vi "GUI.vi"() -> ()   [LabVIEW 2023]
uses:
  <vilib>/Platform/TimedLoop/XDataNode/timing_clust.ctl
  <vilib>/Platform/TimedLoop/XDataNode/nitl_modes.ctl
  <vilib>/Platform/TimedLoop/XDataNode/wakeup.ctl
  <vilib>/Instr/_visa.llb/VISA Configure Serial Port (Instr).vi
  <vilib>/Platform/TimedLoop/XDataNode/XDataNode.xnode
  <vilib>/Platform/TimedLoop/XDataNode/XDNodeRunTimeDep.lvlib
panel:
  out "read buffer":string
  out "Duty":sgl format="%#.4f"
  in  "?":bool
  in  "KD":sgl=0.001 format="%#.4f"
  in  "KI":sgl=0.1 format="%#.4f"
  in  "KP":sgl=1.0 format="%#.4f"
  out "Actual speed":sgl format="%#.1g"
  out "Actual speed":sgl(slide) scale=0.0..3000.0
  out "REV":bool
  out "FWD":bool
  in  "?":bool
  in  "Controller port":refnum<visa-resource-name>
  out "Actual set speed":sgl format="%#.1g"
  out "Throttle set speed":sgl format="%#.0f"
  out "?":T1(graph)
  out "Actual set speed":sgl(slide) scale=0.0..3000.0
  out "Throttle set speed":sgl(slide) scale=0.0..3000.0
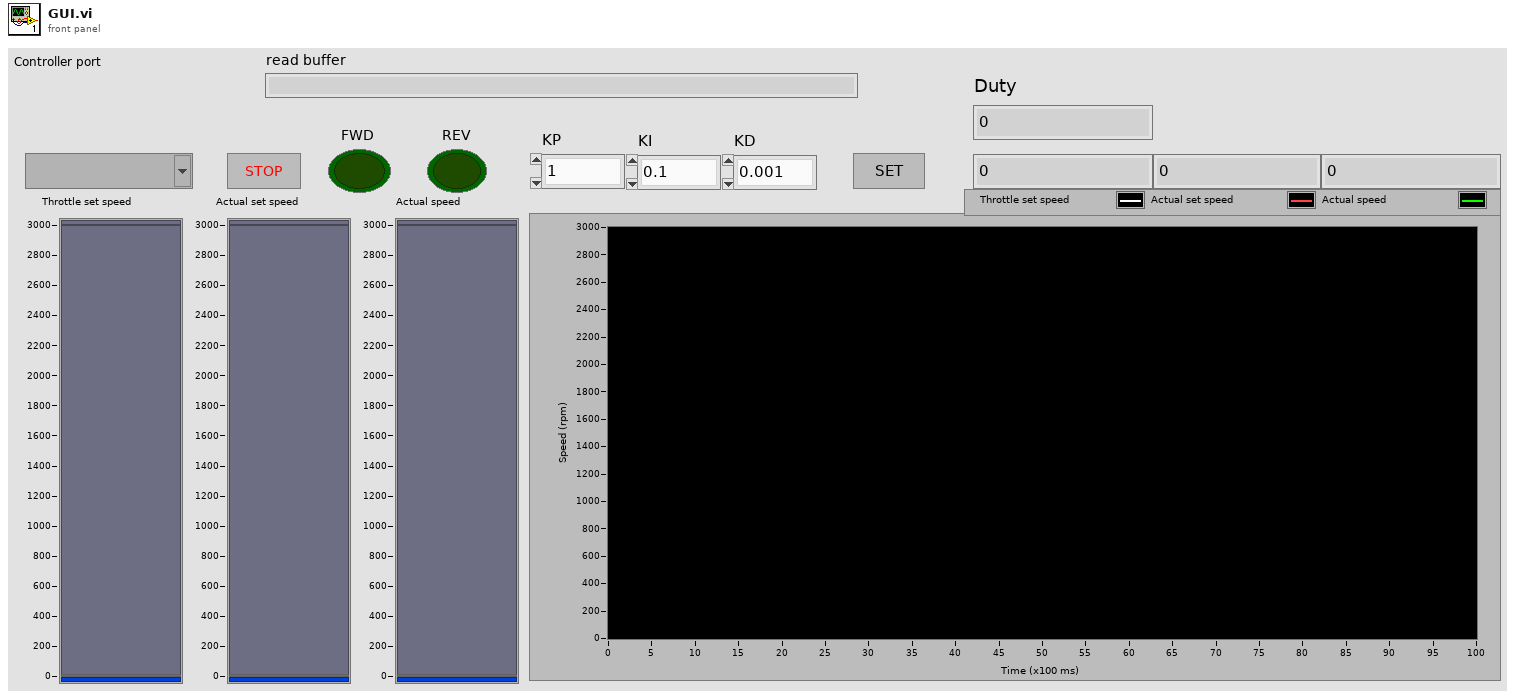
[diagram p1: front panel]
types:
  T1 = cluster{"num_float":sgl, "num_float":sgl, "num_float":sgl}
  T2 = typedef "XDNodeRunTimeDep.lvlib/timing_clust.ctl" = cluster{"Expected End [f-1]":u64, "Actual End [f-1]":u64, "Finished Late? [f-1]":bool, "Expected End [i-1]":u64, "Actual End [i-1]":u64, "Finished Late? [i-1]":bool, "Expected Start [i]":u64, "Actual Start [i]":u64, "Expected Start [f]":u64, "Actual Start [f]":u64, "Source Name":string, "Structure Name":string, "Period":i64, "Deadline":i64, "Offset":i64, "Start":i64, "Priority":i32, "Timeout":i32, "Mode":T3, "Wakeup Reason":T4, "Error":errorcluster, "Source Type":string, "Secondary Source Type":string, "Global End Time":u64, "Global Start Time":u64, "Frame Duration":u64, "Iteration Duration":u64, "Assigned CPU":i32, "I/O Scan Engine Mode":u32}
  T3 = typedef "XDNodeRunTimeDep.lvlib/nitl_modes.ctl" = enum32{"No Change", "Process missed periods, maintain original phase", "Discard missed periods, maintain original phase", "Process missed periods, ignore original phase", "Discard missed periods, ignore original phase"}
  T4 = typedef "XDNodeRunTimeDep.lvlib/wakeup.ctl" = enum32{"Normal", "Aborted", "Asynchronous wakeup", "Timing source error", "Timed loop error", "Timeout"}
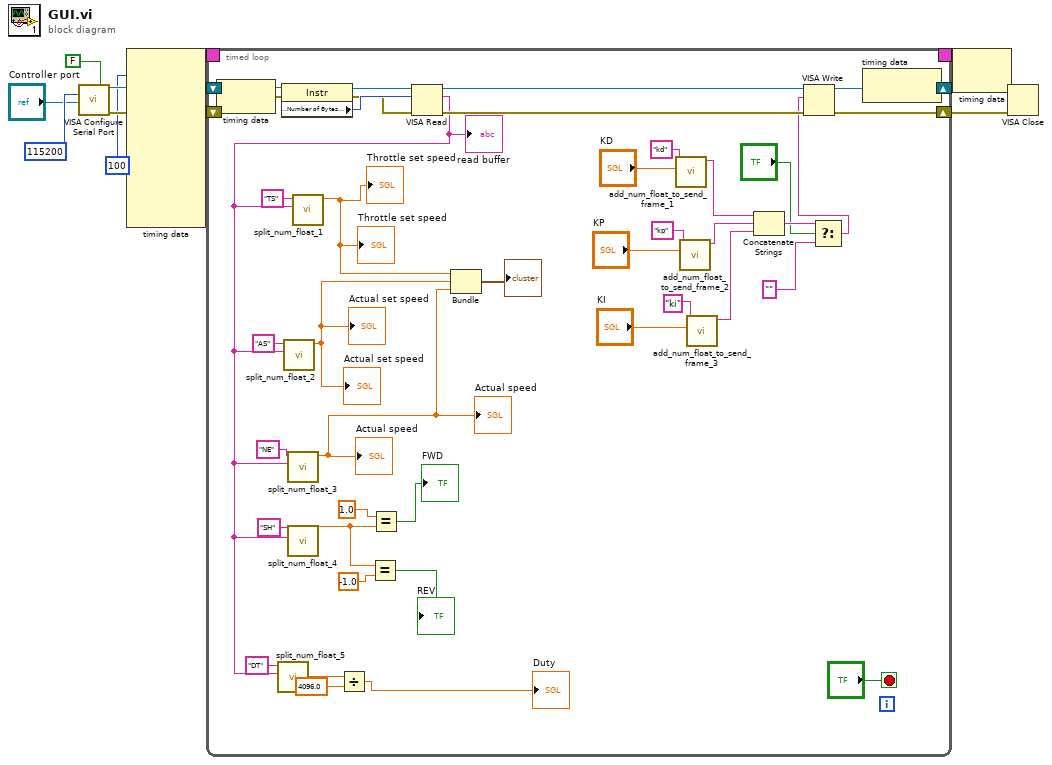
[diagram p0: block diagram]
diagram:
  n1 = call-poly "VISA Configure Serial Port"("VISA resource name"="Controller port", "Enable Termination\nChar (T)"=FALSE ("Enable Termination\nChar (T)"), "baud rate (9600)"=u32 115200) -> ("VISA resource name out"=w10:refnum<visa-resource-name>, "error out"=w9:errorcluster)  [unwired: 11 in]
  n2 = node-c288(i64 100 ("Period")) -> (w6:T2)  [unwired: 9 in]
  n3 = timed-loop {
    timing: w6 -> [_]
    timing-out: [_] -> w5
    shift-right: [w22] -> w8
    shift-left: w10 -> [w46]
    shift-right: [w20] -> w7
    shift-left: w9 -> [w45]
    stop <- "?" stop-if-true
    n4 = node-c288() -> ()  [unwired: 1 in, 1 out]
    n5 = property class="Instr"(reference=w46, error in=w45) -> (reference out=w47:refnum<visa-resource-name>, error out=w44:errorcluster, "Serial Settings:Number of Bytes at Serial Port"=w48:u32)
    n6 = VISA Read(VISA resource name=w47, byte count=w48, error in (no error)=w44) -> (VISA resource name out=w23:refnum<visa-resource-name>, read buffer=w14:string, error out=w21:errorcluster)  [unwired: 1 out]
    "read buffer" <- w14
    n7 = call "split_num_float_5.vi"("read_frame"=w14, "id (2 characters)"="DT") -> ("num_float"=w13:sgl)  [unwired: 9 in]
    n8 = call "split_num_float_2.vi"("read_frame"=w14, "id (2 characters)"="AS") -> ("num_float"=w50:sgl)  [unwired: 9 in]
    "Actual set speed" <- w50
    "Actual set speed" <- w50
    n9 = call "split_num_float_3.vi"("read_frame"=w14, "id (2 characters)"="NE") -> ("num_float"=w33:sgl)  [unwired: 9 in]
    "Actual speed" <- w33
    "Actual speed" <- w33
    n10 = call "split_num_float_4.vi"("read_frame"=w14, "id (2 characters)"="SH") -> ("num_float"=w38:sgl)  [unwired: 9 in]
    n11 = call "split_num_float_1.vi"("read_frame"=w14, "id (2 characters)"="TS") -> ("num_float"=w51:sgl)  [unwired: 9 in]
    "Throttle set speed" <- w51
    "Throttle set speed" <- w51
    n12 = Divide(x=w13, y=sgl 4096.0) -> (x/y=→"Duty":sgl)
    n13 = Equal?(x=w38, y=sgl -1.0) -> (x = y?=→"REV":bool)
    n14 = Equal?(x=sgl 1.0, y=w38) -> (x = y?=→"FWD":bool)
    n15 = Bundle("num_float"=w51, "num_float"=w50, "num_float"=w33) -> (→"?":T1)  [unwired: 1 in]
    n16 = call "add_num_float_to_send_frame_1.vi"("num_float"="KD", "id (2 characters)"="kd") -> ("String"=w26:string)  [unwired: 9 in]
    n17 = call "add_num_float_to_send_frame_2.vi"("num_float"="KP", "id (2 characters)"="kp") -> ("String"=w25:string)  [unwired: 9 in]
    n18 = call "add_num_float_to_send_frame_3.vi"("num_float"="KI", "id (2 characters)"="ki") -> ("String"=w24:string)  [unwired: 9 in]
    n19 = Concatenate Strings(w26, w25, w24) -> (w19:string)
    n20 = Select(t=w19, s="?", f="") -> (s? t:f=w17:string)
    n21 = VISA Write(VISA resource name=w23, write buffer=w17, error in (no error)=w21) -> (VISA resource name out=w22:refnum<visa-resource-name>, error out=w20:errorcluster)  [unwired: 1 out]
    n22 = node-c288() -> ()  [unwired: 1 in, 1 out]
  }
  n23 = node-c288(w5) -> ()  [unwired: 1 out]
  n24 = VISA Close(VISA resource name=w8, error in (no error)=w7) -> ()  [unwired: 1 out]
